vi "Open Library.vi"(6 "Library Path":path=path "", 8 "error in":errorcluster, 11 "Library Icon Data in":refnum<class "Library Icon Data.lvclass">) -> (0 "error out":errorcluster, 3 "Library Icon Data out":refnum<class "Library Icon Data.lvclass">)   [LabVIEW 2020, in "Library Icon Data.lvclass"]
doc: "Opens an Application reference and creates or opens the library at the given path."
uses:
  Library Icon Data.lvclass
  Library Icon Data.lvclass/Library Icon Data.ctl
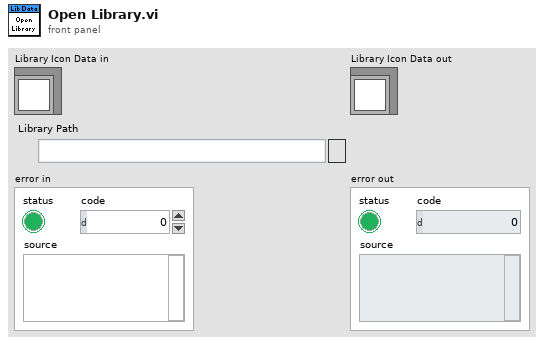
[diagram p1: front panel]
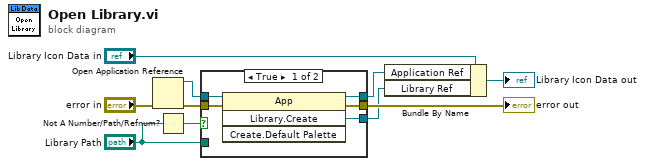
[diagram p0: block diagram]
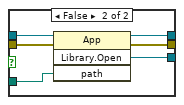
[diagram p2: hidden frame]
diagram:
  n1 = Open Application Reference(8:"error in") -> (0:w10:errorcluster, 3:w7:refnum<vi>)  [unwired: 3 in]
  n2 = Not A Number/Path/Refnum?(number/path/refnum="Library Path") -> (NaN/Path/Refnum?=w2:bool)
  n3 = case shown="True" w2 {
    tunnel: w10 -> [w15 w21]
    tunnel: [w14 w20] -> w8
    tunnel: w7 -> [w13 w19]
    tunnel: [w12 w18] -> w5
    tunnel: [w11 w17] -> w4
    tunnel: "Library Path" -> [_ w16]
    frame True {
      n4 = invoke class="App" method="Library.Create"(reference=w13, error in=w15) -> (reference out=w12:refnum<vi>, error out=w14:errorcluster, "Create Library"=w11:refnum<vi>)  [unwired: 2 in, 1 out]
    }
    frame False {
      n5 = invoke class="App" method="Library.Open"(reference=w19, error in=w21, "path"=w16) -> (reference out=w18:refnum<vi>, error out=w20:errorcluster, "Open Library"=w17:refnum<vi>)  [unwired: 1 in, 1 out]
    }
  }
  "error out" <- w8
  n6 = Bundle By Name(cluster="Library Icon Data in", "Application Ref"=w5, "Library Ref"=w4) -> (→"Library Icon Data out":refnum<class "Library Icon Data.lvclass">)
